vi "Example.vi"() -> ()   [LabVIEW 2020, in "Topas4.lvlib"]
uses:
  Topas4.lvlib
panel:
  in  "Shutter":bool
  out "WL Set Progress":u8(slide) scale=0.0..100.0
  out "WL Set in Prog":bool
  out "Wavelength":dbl
  in  "Wavelength Target":dbl
  in  "Interaction Types":i32(listbox)
  in  "Set Wavelength":bool
  out "error out":errorcluster
  in  "stop":bool
  in  "Serial Number":string
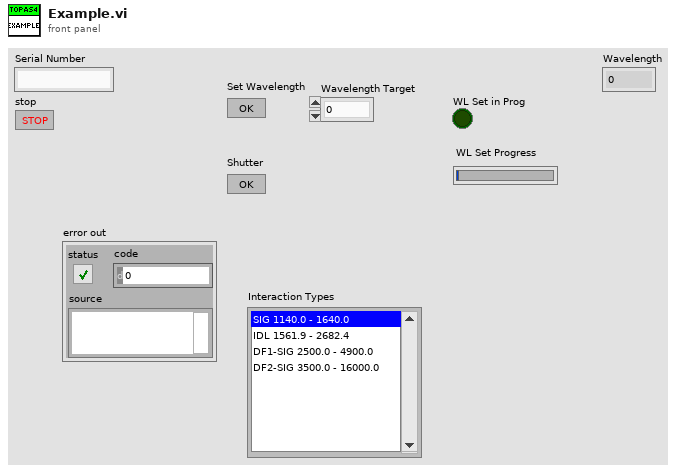
[diagram p1: front panel]
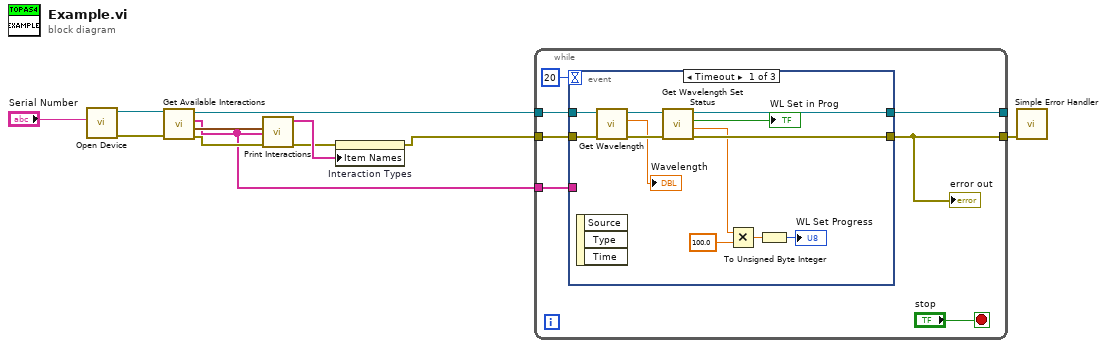
[diagram p0: block diagram]
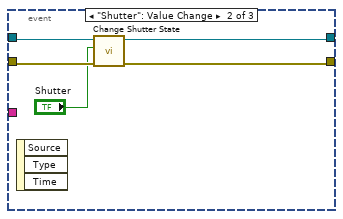
[diagram p2: hidden frame]
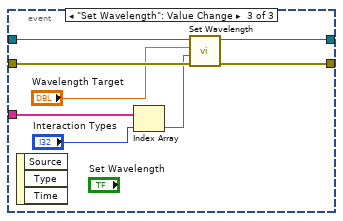
[diagram p3: hidden frame]
diagram:
  n1 = call "Open Device.vi"("Serial Number"="Serial Number") -> ("error out"=w9:errorcluster, "reference out"=w10:refnum<k24>)  [unwired: 9 in]
  n2 = call "Get Available Interactions.vi"("error in"=w9, "reference"=w10) -> ("error out"=w5:errorcluster, "Interaction Ranges"=w6:cluster{"From":dbl, "To":dbl}[], "Interaction Types"=w1:string[], "reference out"=w8:refnum<k24>)  [unwired: 6 in]
  n3 = call "Print Interactions.vi"("error in (no error)"=w5, "Interaction Ranges"=w6, "Interaction Types"=w1) -> ("error out"=w3:errorcluster, "Array"=w4:string[])  [unwired: 7 in]
  n4 = property on="Interaction Types" class="LstBox (strict)"(error in=w3, "Item Names"=w4) -> (error out=w2:errorcluster)  [unwired: 1 in, 1 out]
  n5 = while {
    tunnel: w8 -> [w17]
    tunnel: [w16] -> w7
    tunnel: w2 -> [w14]
    tunnel: [w13] -> _
    tunnel: w1 -> [w12]
    stop <- "stop" stop-if-true
    n6 = event shown="[0] Timeout" {
      selector: _ -> [_ _ _]
      dyn-events: _ -> [_ _ _]
      timeout: 20 -> [_ _ _]
      tunnel: w17 -> [w30 w35 w43]
      tunnel: [w26 w33 w41] -> w16
      tunnel: w14 -> [w27 w34 w42]
      tunnel: [w24 w32 w40] -> w13
      tunnel: w12 -> [_ _ w38]
      event Timeout {
        n7 = event-data() -> ()  [unwired: 1 in, 3 out]
        n8 = call "Get Wavelength.vi"("error in"=w27, "reference"=w30) -> ("error out"=w29:errorcluster, "GetOutputWavelength"=→"Wavelength":dbl, "reference out"=w25:refnum<k24>)  [unwired: 7 in]
        n9 = call "Get Wavelength Set Status.vi"("error in"=w29, "reference"=w25) -> ("error out"=w26:errorcluster, "WavelengthSettingCompletionPart"=w21:dbl, "IsWavelengthSettingInProgress"=→"WL Set in Prog":bool, "reference out"=w24:refnum<k24>)  [unwired: 6 in]
        n10 = Multiply(x=w21, y=100.0) -> (x*y=w22:dbl)
        n11 = To Unsigned Byte Integer(number=w22) -> (unsigned 8bit integer=→"WL Set Progress":u8)
      }
      event "Shutter": Value Change {
        n12 = event-data() -> ()  [unwired: 1 in, 3 out]
        n13 = call "Change Shutter State.vi"("error in"=w34, "open"="Shutter", "reference"=w35) -> ("error out"=w33:errorcluster, "reference out"=w32:refnum<k24>)  [unwired: 7 in]
      }
      event "Set Wavelength": Value Change {
        n14 = event-data() -> ()  [unwired: 1 in, 3 out]
        n15 = Index Array(array=w38, index="Interaction Types") -> (element=w36:string)
        n16 = call "Set Wavelength.vi"("error in"=w42, "Interaction Type"=w36, "Wavelength"="Wavelength Target", "reference"=w43) -> ("error out"=w41:errorcluster, "reference out"=w40:refnum<k24>)  [unwired: 6 in]
      }
    }
    "error out" <- w16
  }
  n17 = call <vilib>:"Simple Error Handler.vi"("error in (no error)"=w7) -> ()  [unwired: 4 in, 5 out]
